vi "Menu.Sequeunce.Execute.vi"(8 "error in (no error)":errorcluster, 9 "Coords":T1, 10 "ItemPath":string, 11 "Cluster in":T2) -> (0 "error out":errorcluster, 3 "Cluster out":T2)   [LabVIEW 2013, in "Simple Sequence Editor.lvlib"]
uses:
  Simple Sequence Editor.lvlib
  Types/StateVariables.ctl
  Types/ChannelProperties.ctl
  <vilib>/Utility/miscctls.llb/LVPoint32TypeDef.ctl
  <vilib>/Utility/miscctls.llb/LVBoundsTypeDef.ctl
  Constants.vi
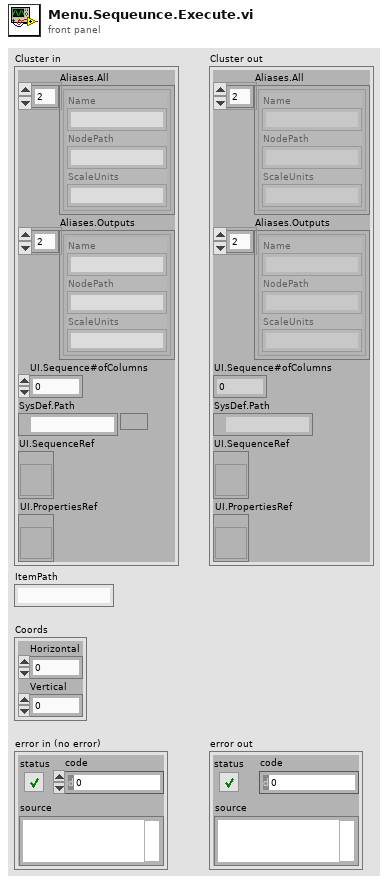
[diagram p1: front panel]
types:
  T1 = typedef "LVPoint32TypeDef.ctl" = cluster{"Horizontal":i32, "Vertical":i32}
  T2 = typedef "Simple Sequence Editor.lvlib/StateVariables.ctl" = cluster{"Aliases.All":T3[], "Aliases.Outputs":T3[], "UI.Sequence#ofColumns":i32, "SysDef.Path":path, "UI.SequenceRef":refnum<vi>, "UI.PropertiesRef":refnum<vi>}
  T3 = typedef "Simple Sequence Editor.lvlib/ChannelProperties.ctl" = cluster{"Name":string, "NodePath":string, "ScaleUnits":string}
  T4 = typedef "LVRowAndColumnTypeDef.ctl" = cluster{"Row":i32, "Column":i32}
  T5 = typedef "LVBoundsTypeDef.ctl" = cluster{"Width":u32, "Height":u32}
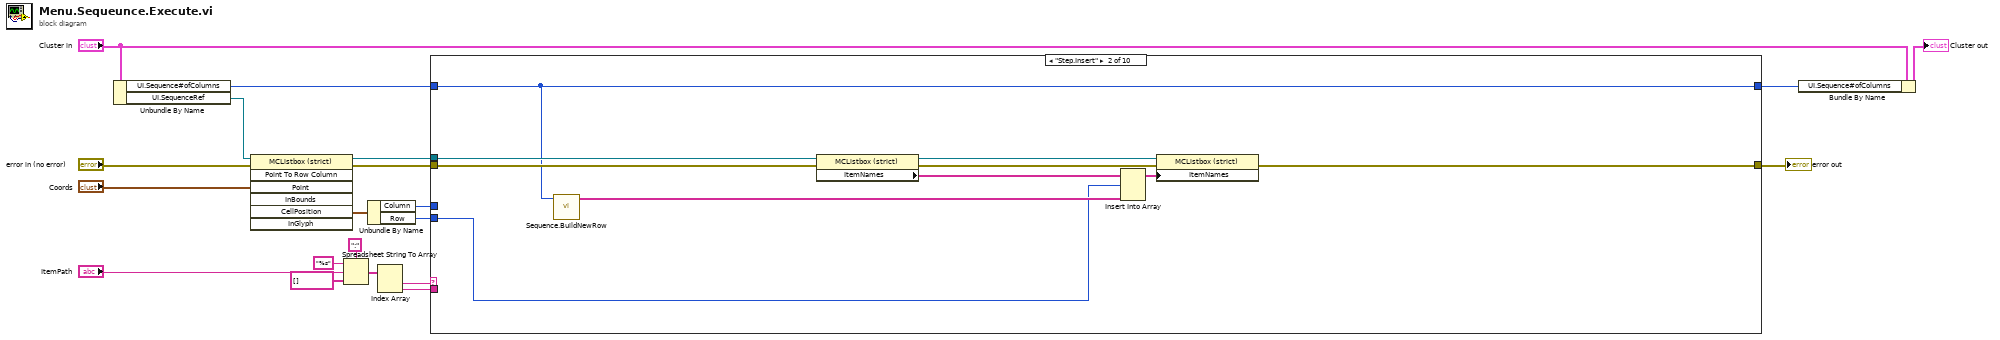
[diagram p0: block diagram]
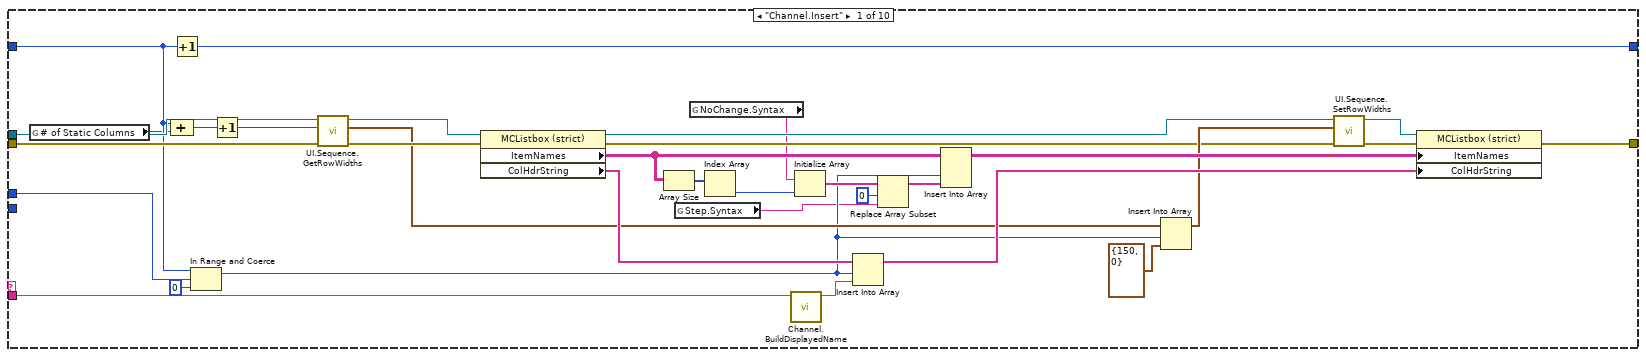
[diagram p2: hidden frame]
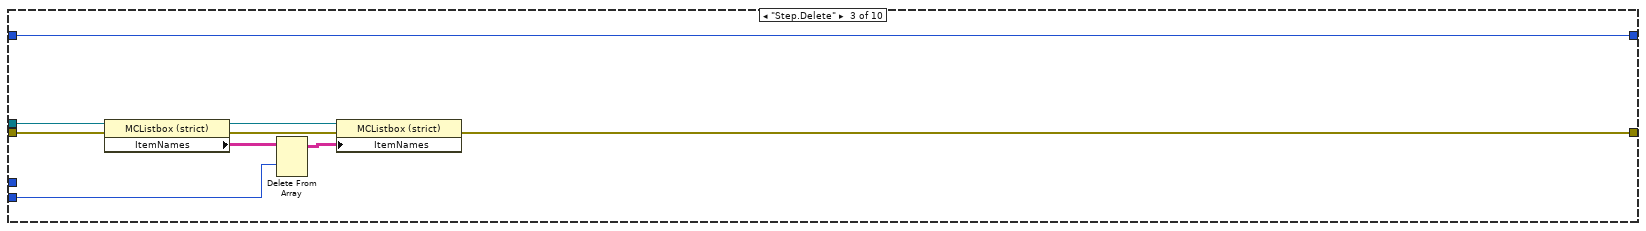
[diagram p3: hidden frame]
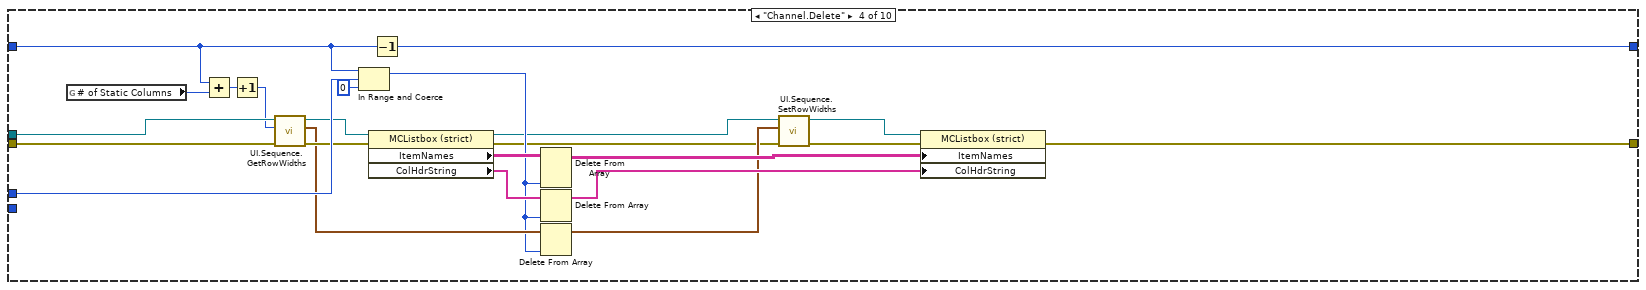
[diagram p4: hidden frame]
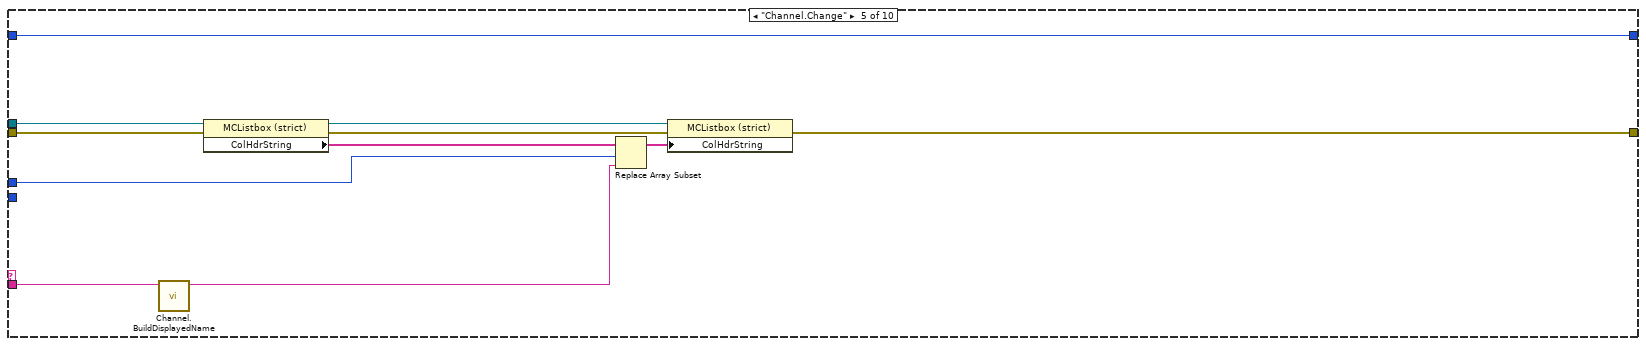
[diagram p5: hidden frame]
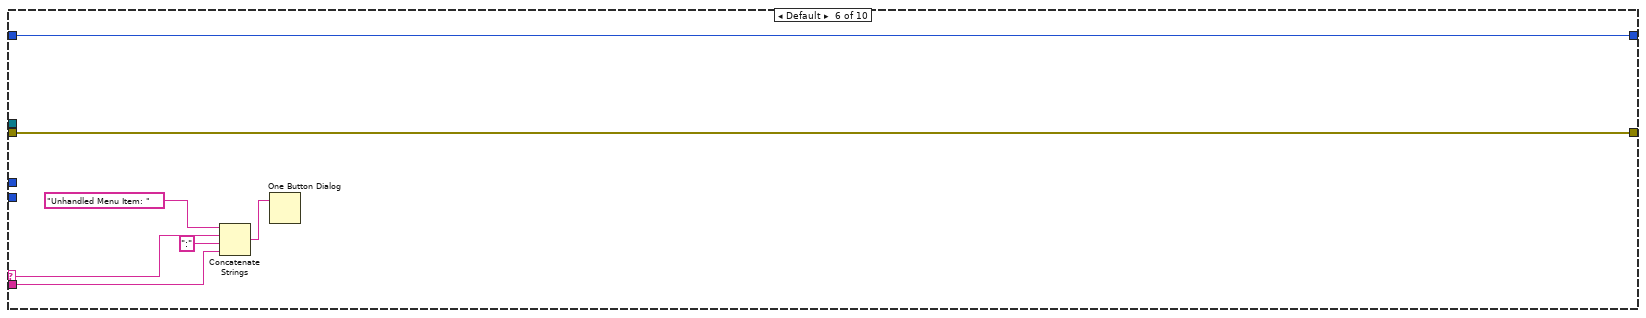
[diagram p6: hidden frame]
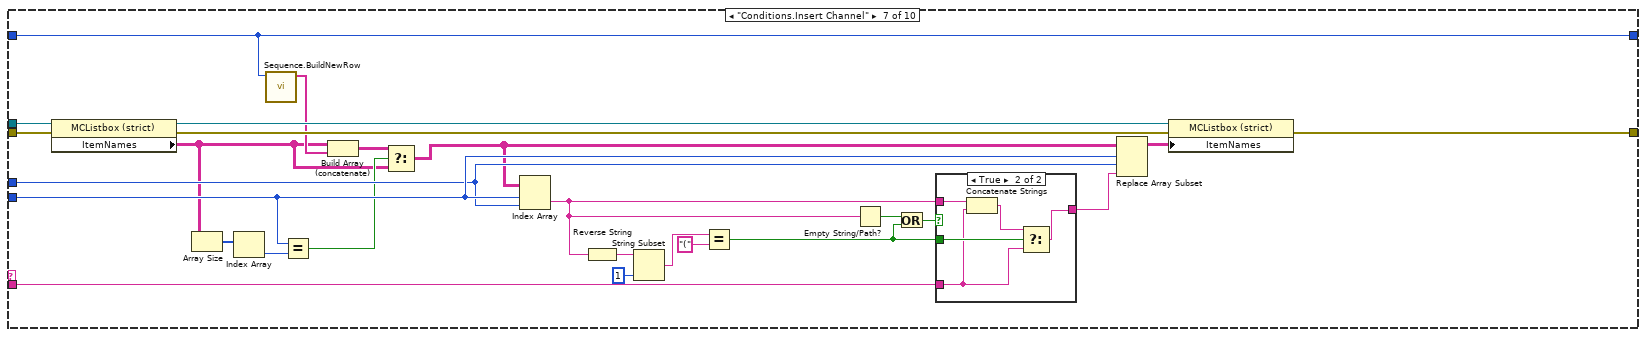
[diagram p7: hidden frame]
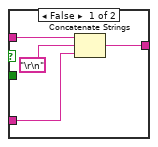
[diagram p8: hidden frame]
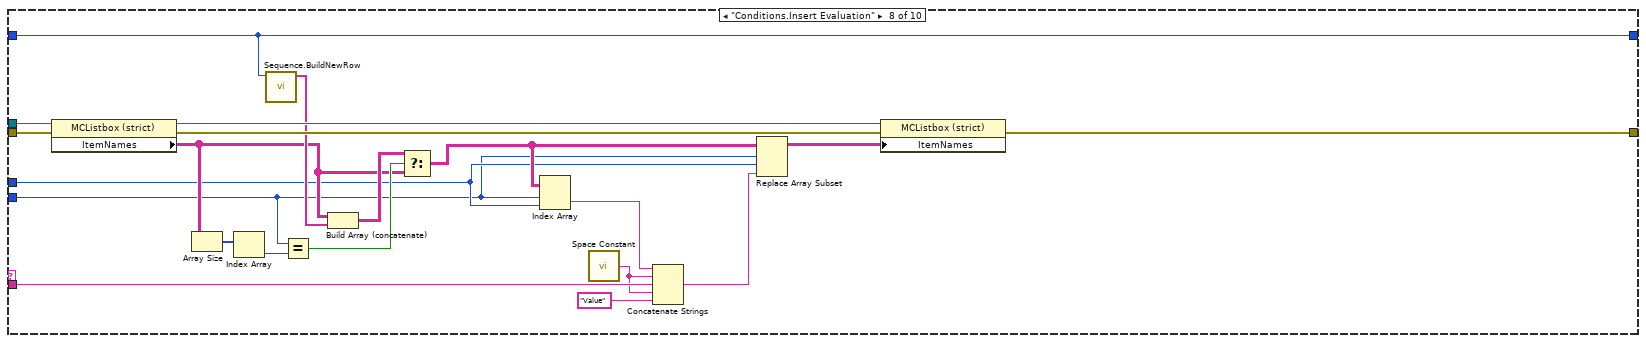
[diagram p9: hidden frame]
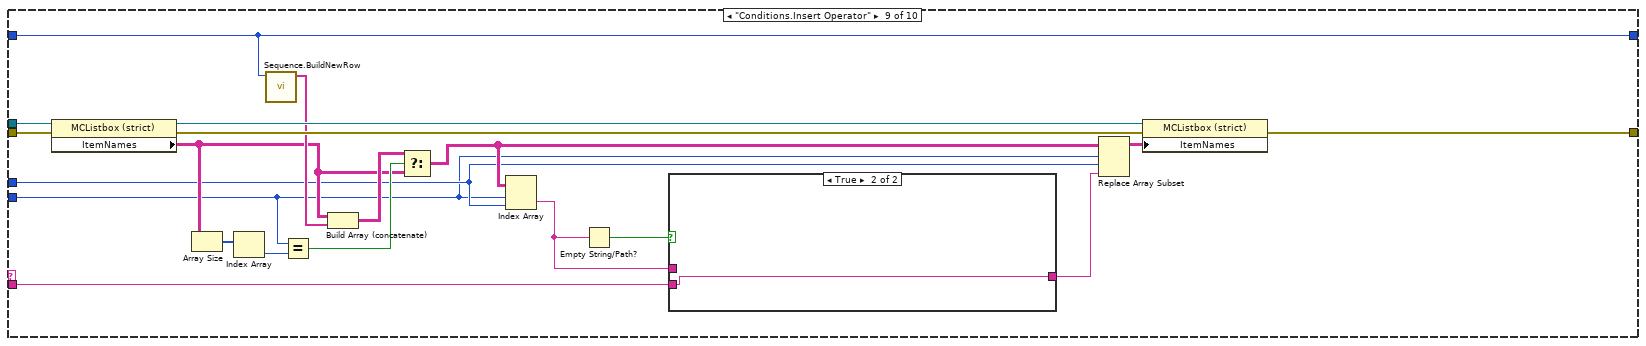
[diagram p10: hidden frame]
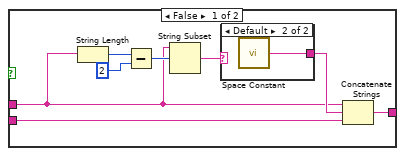
[diagram p11: hidden frame]
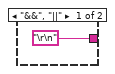
[diagram p12: hidden frame]
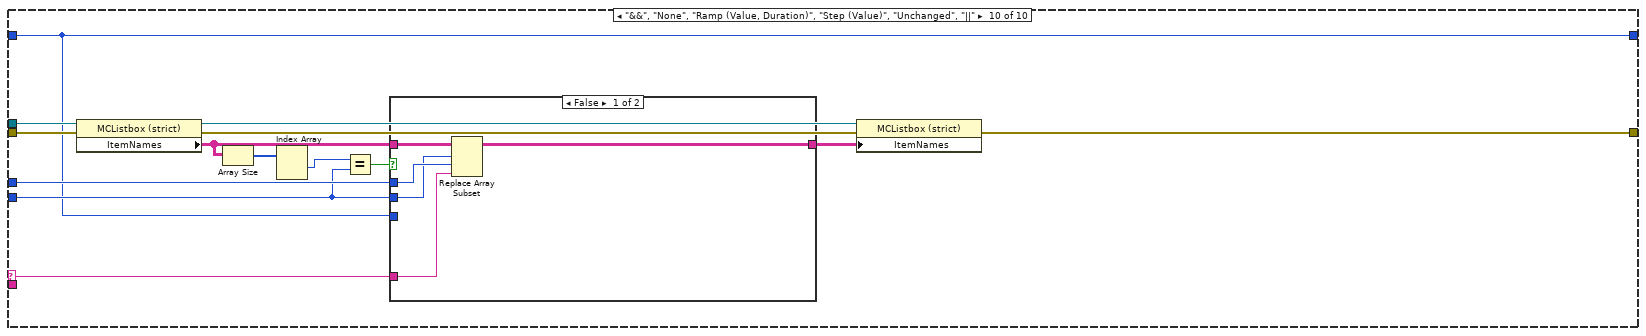
[diagram p13: hidden frame]
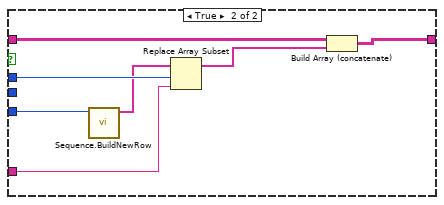
[diagram p14: hidden frame]
diagram:
  n1 = Unbundle By Name("Cluster in") -> ("UI.Sequence#ofColumns"=w11:i32, "UI.SequenceRef"=w8:refnum<vi>)
  n2 = invoke class="MCListbox (strict)" method="Point To Row Column"(reference=w8, error in="error in (no error)", "Point"="Coords") -> (reference out=w13:refnum<vi>, error out=w14:errorcluster, "CellPosition"=w10:T4)  [unwired: 4 in, 4 out]
  n3 = Spreadsheet String To Array(delimiter (Tab)=":", format string="%s", spreadsheet string="ItemPath", array type (2D Dbl)=string[] []) -> (array=w6:string[])
  n4 = Unbundle By Name(w10) -> ("Column"=w12:i32, "Row"=w1:i32)
  n5 = Index Array(array=w6) -> (element #1=w7:string, element #2=w15:string)  [unwired: 2 in]
  n6 = case shown="\"Step.Insert\"" w7 {
    selector: w7 -> [_ _ _ _ _ w111 _ _ _ w203]
    tunnel: w11 -> [w35 w54 w64 w79 w106 w113 w130 w162 w182 w201]
    tunnel: w12 -> [w53 _ _ w95 w99 _ w124 w152 w173 w209]
    tunnel: w13 -> [w38 w59 w68 w86 w100 _ w139 w169 w189 w213]
    tunnel: w14 -> [w40 w60 w69 w88 w101 w112 w138 w168 w188 w214]
    tunnel: w15 -> [w42 _ _ _ w97 w109 w134 w164 w184 _]
    tunnel: [w22 w61 w70 w73 w98 w112 w136 w166 w186 w202] -> w17
    tunnel: [w33 w54 w64 w93 w106 w113 w130 w162 w182 w201] -> w20
    tunnel: w1 -> [_ w55 w65 _ _ _ w127 w151 w172 w205]
    frame "Channel.Insert" {
      n7 = global read "Constants.vi" "# of Static Columns"() -> (w34:u32)
      n8 = Compound Arithmetic op=ADD(w35, w34) -> (w36:u32)
      n9 = Increment(x=w35) -> (x+1=w33:i32)
      n10 = In Range and Coerce(upper limit=w35, x=w53, lower limit=0) -> (coerced(x)=w30:i32)  [unwired: 1 out]
      n11 = Increment(x=w36) -> (x+1=w28:u32)
      n12 = call "UI.Sequence.GetRowWidths.vi"("error in (no error)"=w40, "Numeric"=w28, "MulticolumnListbox in"=w38) -> ("error out"=w39:errorcluster, "Array"=w31:T5[], "MulticolumnListbox out"=w37:refnum<vi>)  [unwired: 6 in]
      n13 = property class="MCListbox (strict)"(reference=w37, error in=w39) -> (reference out=w23:refnum<vi>, error out=w26:errorcluster, "ItemNames"=w50:string[][], "ColHdrString"=w45:string[])
      n14 = Array Size(array=w50) -> (size(s)=w51:i32[])
      n15 = global read "Constants.vi" "Step.Syntax"() -> (w27:string)
      n16 = global read "Constants.vi" "NoChange.Syntax"() -> (w21:string)
      n17 = Index Array(array=w51) -> (element=w49:i32)  [unwired: 1 in]
      n18 = call "Channel.BuildDisplayedName.vi"("String in"=w42) -> ("String out"=w41:string)  [unwired: 10 in]
      n19 = Initialize Array(w21, w49) -> (w48:string[])
      n20 = Insert Into Array(array=w45, index=w30, new element=w41) -> (w46:string[])
      n21 = Replace Array Subset(array=w48, new element=w27, index=0) -> (w44:string[])
      n22 = Insert Into Array(array=w50, index (col)=w30, new element=w44) -> (w47:string[][])  [unwired: 1 in]
      n23 = Insert Into Array(array=w31, index=w30, new element=T5 {"Width"=150, "Height"=0} ("new element/subarray")) -> (w32:T5[])
      n24 = call "UI.Sequence.SetRowWidths.vi"("error in (no error)"=w26, "Array"=w32, "MulticolumnListbox in"=w23) -> ("error out"=w25:errorcluster, "MulticolumnListbox out"=w24:refnum<vi>)  [unwired: 7 in]
      n25 = property class="MCListbox (strict)"(reference=w24, error in=w25, "ItemNames"=w47, "ColHdrString"=w46) -> (error out=w22:errorcluster)  [unwired: 1 out]
    }
    frame "Step.Insert" {
      n26 = call "Sequence.BuildNewRow.vi"("UI.Sequence#ofColumns"=w54) -> ("New Array"=w58:string[])  [unwired: 10 in]
      n27 = property class="MCListbox (strict)"(reference=w59, error in=w60) -> (reference out=w56:refnum<vi>, error out=w57:errorcluster, "ItemNames"=w63:string[][])
      n28 = Insert Into Array(array=w63, index (row)=w55, new element=w58) -> (w62:string[][])  [unwired: 1 in]
      n29 = property class="MCListbox (strict)"(reference=w56, error in=w57, "ItemNames"=w62) -> (error out=w61:errorcluster)  [unwired: 1 out]
    }
    frame "Step.Delete" {
      n30 = property class="MCListbox (strict)"(reference=w68, error in=w69) -> (reference out=w66:refnum<vi>, error out=w67:errorcluster, "ItemNames"=w72:string[][])
      n31 = Delete From Array(array=w72, index (row)=w65) -> (array with subset deleted=w71:string[][])  [unwired: 2 in, 1 out]
      n32 = property class="MCListbox (strict)"(reference=w66, error in=w67, "ItemNames"=w71) -> (error out=w70:errorcluster)  [unwired: 1 out]
    }
    frame "Channel.Delete" {
      n33 = global read "Constants.vi" "# of Static Columns"() -> (w81:u32)
      n34 = Add(x=w79, y=w81) -> (x+y=w80:u32)
      n35 = Increment(x=w80) -> (x+1=w78:u32)
      n36 = call "UI.Sequence.GetRowWidths.vi"("error in (no error)"=w88, "Numeric"=w78, "MulticolumnListbox in"=w86) -> ("error out"=w87:errorcluster, "Array"=w84:T5[], "MulticolumnListbox out"=w85:refnum<vi>)  [unwired: 6 in]
      n37 = In Range and Coerce(upper limit=w79, x=w95, lower limit=0) -> (coerced(x)=w83:i32)  [unwired: 1 out]
      n38 = property class="MCListbox (strict)"(reference=w85, error in=w87) -> (reference out=w74:refnum<vi>, error out=w77:errorcluster, "ItemNames"=w92:string[][], "ColHdrString"=w89:string[])
      n39 = Decrement(x=w79) -> (x-1=w93:i32)
      n40 = Delete From Array(array=w92, index (col)=w83) -> (array with subset deleted=w91:string[][])  [unwired: 2 in, 1 out]
      n41 = Delete From Array(array=w89, index=w83) -> (array with subset deleted=w90:string[])  [unwired: 1 in, 1 out]
      n42 = Delete From Array(array=w84, index=w83) -> (array with subset deleted=w82:T5[])  [unwired: 1 in, 1 out]
      n43 = call "UI.Sequence.SetRowWidths.vi"("error in (no error)"=w77, "Array"=w82, "MulticolumnListbox in"=w74) -> ("error out"=w76:errorcluster, "MulticolumnListbox out"=w75:refnum<vi>)  [unwired: 7 in]
      n44 = property class="MCListbox (strict)"(reference=w75, error in=w76, "ItemNames"=w91, "ColHdrString"=w90) -> (error out=w73:errorcluster)  [unwired: 1 out]
    }
    frame "Channel.Change" {
      n45 = call "Channel.BuildDisplayedName.vi"("String in"=w97) -> ("String out"=w96:string)  [unwired: 10 in]
      n46 = property class="MCListbox (strict)"(reference=w100, error in=w101) -> (reference out=w105:refnum<vi>, error out=w104:errorcluster, "ColHdrString"=w102:string[])
      n47 = Replace Array Subset(array=w102, new element=w96, index=w99) -> (w103:string[])
      n48 = property class="MCListbox (strict)"(reference=w105, error in=w104, "ColHdrString"=w103) -> (error out=w98:errorcluster)  [unwired: 1 out]
    }
    frame Default {
      n49 = Concatenate Strings("Unhandled Menu Item: " ("message"), w111, ":" ("string"), w109) -> (w107:string)
      n50 = One Button Dialog(message=w107) -> ()  [unwired: 1 in, 1 out]
    }
    frame "Conditions.Insert Channel" {
      n51 = property class="MCListbox (strict)"(reference=w139, error in=w138) -> (reference out=w135:refnum<vi>, error out=w137:errorcluster, "ItemNames"=w122:string[][])
      n52 = Array Size(array=w122) -> (size(s)=w129:i32[])
      n53 = Index Array(array=w129) -> (element=w128:i32)  [unwired: 1 in]
      n54 = call "Sequence.BuildNewRow.vi"("UI.Sequence#ofColumns"=w130) -> ("New Array"=w126:string[])  [unwired: 10 in]
      n55 = Equal?(x=w127, y=w128) -> (x = y?=w123:bool)
      n56 = Build Array (concatenate)(w122, w126) -> (w125:string[][])
      n57 = Select(t=w125, s=w123, f=w122) -> (s? t:f=w119:string[][])
      n58 = Index Array(array=w119, index (row)=w127, index (col)=w124) -> (element=w115:string)
      n59 = Reverse String(1:w115) -> (0:w117:string)
      n60 = String Subset(string=w117, length (rest)=1 ("length (rest)")) -> (substring=w114:string)  [unwired: 1 in]
      n61 = Equal?(x=w114, y="(") -> (x = y?=w118:bool)
      n62 = Empty String/Path?(string/path=w115) -> (empty?=w133:bool)
      n63 = Or(x=w133, y=w118) -> (x .or. y?=w120:bool)
      n64 = case shown="True" w120 {
        tunnel: w115 -> [w143 w147]
        tunnel: w134 -> [w142 w146]
        tunnel: [w140 w145] -> w132
        tunnel: w118 -> [_ w148]
        frame False {
          n65 = Concatenate Strings(w143, "\r\n", w142) -> (w140:string)
        }
        frame True {
          n66 = Concatenate Strings(w147, w146) -> (w144:string)
          n67 = Select(t=w144, s=w148, f=w146) -> (s? t:f=w145:string)
        }
      }
      n68 = Replace Array Subset(array=w119, new element=w132, index (row)=w127, index (col)=w124) -> (w131:string[][])
      n69 = property class="MCListbox (strict)"(reference=w135, error in=w137, "ItemNames"=w131) -> (error out=w136:errorcluster)  [unwired: 1 out]
    }
    frame "Conditions.Insert Evaluation" {
      n70 = property class="MCListbox (strict)"(reference=w169, error in=w168) -> (reference out=w165:refnum<vi>, error out=w167:errorcluster, "ItemNames"=w156:string[][])
      n71 = Array Size(array=w156) -> (size(s)=w161:i32[])
      n72 = Index Array(array=w161) -> (element=w160:i32)  [unwired: 1 in]
      n73 = call "Sequence.BuildNewRow.vi"("UI.Sequence#ofColumns"=w162) -> ("New Array"=w159:string[])  [unwired: 10 in]
      n74 = Equal?(x=w151, y=w160) -> (x = y?=w157:bool)
      n75 = Build Array (concatenate)(w156, w159) -> (w158:string[][])
      n76 = Select(t=w158, s=w157, f=w156) -> (s? t:f=w153:string[][])
      n77 = Index Array(array=w153, index (row)=w151, index (col)=w152) -> (element=w149:string)
      n78 = call <vilib>:"Space Constant.vi"() -> ("String"=w150:string)
      n79 = Concatenate Strings(w149, w150, w164, w150, "Value" ("string")) -> (w155:string)
      n80 = Replace Array Subset(array=w153, new element=w155, index (row)=w151, index (col)=w152) -> (w163:string[][])
      n81 = property class="MCListbox (strict)"(reference=w165, error in=w167, "ItemNames"=w163) -> (error out=w166:errorcluster)  [unwired: 1 out]
    }
    frame "Conditions.Insert Operator" {
      n82 = property class="MCListbox (strict)"(reference=w189, error in=w188) -> (reference out=w185:refnum<vi>, error out=w187:errorcluster, "ItemNames"=w176:string[][])
      n83 = Array Size(array=w176) -> (size(s)=w181:i32[])
      n84 = Index Array(array=w181) -> (element=w180:i32)  [unwired: 1 in]
      n85 = call "Sequence.BuildNewRow.vi"("UI.Sequence#ofColumns"=w182) -> ("New Array"=w179:string[])  [unwired: 10 in]
      n86 = Equal?(x=w172, y=w180) -> (x = y?=w177:bool)
      n87 = Build Array (concatenate)(w176, w179) -> (w178:string[][])
      n88 = Select(t=w178, s=w177, f=w176) -> (s? t:f=w174:string[][])
      n89 = Index Array(array=w174, index (row)=w172, index (col)=w173) -> (element=w171:string)
      n90 = Empty String/Path?(string/path=w171) -> (empty?=w170:bool)
      n91 = case shown="True" w170 {
        tunnel: w184 -> [w197 w200]
        tunnel: [w196 w200] -> w175
        tunnel: w171 -> [w190 _]
        frame False {
          n92 = String Length(string=w190) -> (length=w195:i32)
          n93 = Subtract(x=w195, y=2) -> (x-y=w194:i32)
          n94 = String Subset(string=w190, offset (0)=w194) -> (substring=w192:string)  [unwired: 1 in]
          n95 = case shown="Default" w192 {
            tunnel: ["\r\n" w199] -> w191
            frame "&&", "||" {
            }
            frame Default {
              n96 = call <vilib>:"Space Constant.vi"() -> ("String"=w199:string)
            }
          }
          n97 = Concatenate Strings(w190, w191, w197) -> (w196:string)
        }
        frame True {
        }
      }
      n98 = Replace Array Subset(array=w174, new element=w175, index (row)=w172, index (col)=w173) -> (w183:string[][])
      n99 = property class="MCListbox (strict)"(reference=w185, error in=w187, "ItemNames"=w183) -> (error out=w186:errorcluster)  [unwired: 1 out]
    }
    frame "&&", "None", "Ramp (Value, Duration)", "Step (Value)", "Unchanged", "||" {
      n100 = property class="MCListbox (strict)"(reference=w213, error in=w214) -> (reference out=w211:refnum<vi>, error out=w212:errorcluster, "ItemNames"=w208:string[][])
      n101 = Array Size(array=w208) -> (size(s)=w207:i32[])
      n102 = Index Array(array=w207) -> (element #1=w206:i32)  [unwired: 2 in, 1 out]
      n103 = Equal?(x=w206, y=w205) -> (x = y?=w204:bool)
      n104 = case shown="False" w204 {
        tunnel: [w219 w225] -> w210
        tunnel: w209 -> [w218 w224]
        tunnel: w208 -> [w217 w226]
        tunnel: w205 -> [w216 _]
        tunnel: w201 -> [_ w221]
        tunnel: w203 -> [w215 w223]
        frame False {
          n105 = Replace Array Subset(array=w217, new element=w215, index (row)=w216, index (col)=w218) -> (w219:string[][])
        }
        frame True {
          n106 = call "Sequence.BuildNewRow.vi"("UI.Sequence#ofColumns"=w221) -> ("New Array"=w220:string[])  [unwired: 10 in]
          n107 = Replace Array Subset(array=w220, new element=w223, index=w224) -> (w222:string[])
          n108 = Build Array (concatenate)(w226, w222) -> (w225:string[][])
        }
      }
      n109 = property class="MCListbox (strict)"(reference=w211, error in=w212, "ItemNames"=w210) -> (error out=w202:errorcluster)  [unwired: 1 out]
    }
  }
  "error out" <- w17
  n110 = Bundle By Name(cluster="Cluster in", "UI.Sequence#ofColumns"=w20) -> (→"Cluster out":T2)
